vi "Dispense X Gallon at Y Flowrate.vi"(0 "Gallon Target":dbl=10.72, 1 "Equipment":T3={"MW100"="MW100", "AG34970"="A-34972A", "WT210"="A-34972A"}, 5 "GPM Target":dbl=3.0, 11 "Error In":errorcluster, 12 "Test Condition":T5=enum."SRK500,Station1,5GPM FR", 13 "Ctl Refnum":refnum<vi>) -> (6 "M*(Gallons)":dbl, 8 "ToutMax":dbl, 10 "ToutMin":dbl, 14 "POWER Ref":refnum<vi>, 15 "Error Out":errorcluster)   [LabVIEW 2013]
uses:
  Utility/Custom Pallet Controls/Chart.ctl
  Type Definitions/PowerElements.ctl
  Type Definitions/EquipReferences.ctl
  Type Definitions/HEWH Tank Indicator.ctl
  Type Definitions/TestedFlowratesScenarios.ctl
  Utility/Custom Pallet Controls/Timer.ctl
  Type Definitions/PowerData.ctl
  Type Definitions/User Controls.ctl
  Type Definitions/HEWH Output Information.ctl
  <vilib>/Platform/fileVersionInfo.llb/FileVersionInformation.ctl
  Type Definitions/Agilent Cluster.ctl
  Type Definitions/Draw Pattern Setup.ctl
  Type Definitions/PreDraw.ctl
  Type Definitions/Custom Test.ctl
  Type Definitions/Custom Test - Conditions.ctl
  Type Definitions/Termination Condition Cluster.ctl
  Utility/Custom Pallet Controls/DBL.ctl
  Type Definitions/ChannelSettings.ctl
  Type Definitions/Intellfaucet Mode.ctl
panel:
  out "Gather Data Timer":dbl format="%.2f"
  out "Loop Time":dbl
  out "PowerData":T1={"Voltage (Volts)"=236.2, "Current (Amps)"=17.749, "Power (Watts)"=4192.0, "WattHours (Wh)"=0.0, "TC Tree (AVG)"=0.0, "Flow Rate (GPM)"=0.0, "Gallons (Gal)"=0.0, "RTD Out (Deg F)"=0.0, "TC Down"=0.0}
  out "Elapsed Time":T2 format="%<%H:%M:%S>t"
  in  "Tab Control":enum32{"Page 1", "Page 2"}(tab)
  in  "Equipment 2":T3={"MW100"="COM1", "AG34970"="MW100", "WT210"="A-34972A"}
  out "Flow":dbl=3.8899999999999997
  out "String":string
  out "POWER":T4
  out "Dispensed Gallons":dbl
  in  "Gallon Target Value":dbl format="%#_13g"
  in  "GPM Target Value":dbl format="%#_13g"
  in  "Configuration":T5=enum."SRK500,Station1,5GPM FR"
  in  "OK":bool
  out "Tank Display":T6 {"TC6" format="%.2g"; "TIN" format="%.2g"; "TOUT" format="%.2g"; "Mean" format="%.2f"; "Std Dev" format="%.2f"; "TC5" format="%.2g"; "TC4" format="%.2g"; "TC3" format="%.2g"; "TC2" format="%.2g"; "TC1" format="%.2g"}
  out "Flow Chart":T7
  out "MW100":refnum<visa-resource-name>="MW100"
  out "Current Draw Start Time":dbl format="%.2f"
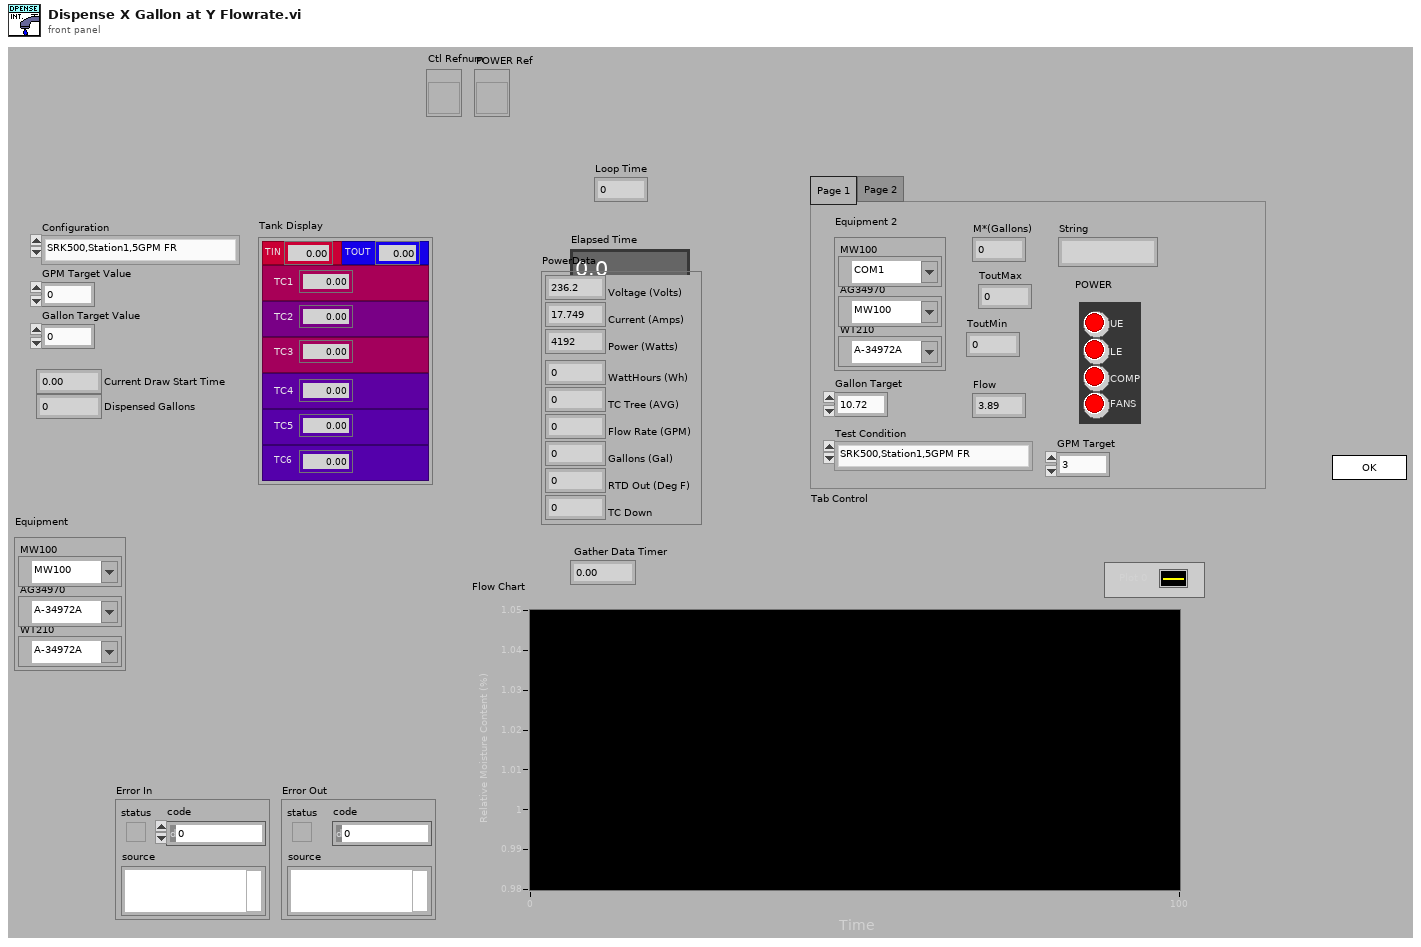
[diagram p1: front panel]
types:
  T1 = typedef "PowerData.ctl" = cluster{"Voltage (Volts)":dbl, "Current (Amps)":dbl, "Power (Watts)":dbl, "WattHours (Wh)":dbl, "TC Tree (AVG)":dbl, "Flow Rate (GPM)":dbl, "Gallons (Gal)":dbl, "RTD Out (Deg F)":dbl, "TC Down":dbl}
  T2 = typedef "Timer.ctl" = dbl
  T3 = typedef "EquipReferences.ctl" = cluster{"MW100":refnum<visa-resource-name>, "AG34970":refnum<visa-resource-name>, "WT210":refnum<visa-resource-name>}
  T4 = typedef "PowerElements.ctl" = cluster{"UE":bool, "LE":bool, "COMP":bool, "FANS":bool}
  T5 = typedef "TestedFlowratesScenarios.ctl" = enum16{"DRK500,Station1", "DRK375,Lab", "SRK500,Station1,5GPM FR", "DRK375,STATION3,1/2\"HOSE", "DRK500,Station1,downspout", "DRK375,Station3,thruEcocute", "DRK375,Station3,purge", "Build2,2B,Purge", "Global, Purge", "Global, Tank", "DRK250"}
  T6 = typedef "HEWH Tank Indicator.ctl" = cluster{"TC1-D":bool, "TC2-D":bool, "TC3-D":bool, "TC4-D":bool, "TC5-D":bool, "RTD_IN":bool, "RTDOUT":bool, "TC1":dbl, "TC2":dbl, "TC3":dbl, "TC4":dbl, "TC5":dbl, "TIN":dbl, "TOUT":dbl, "Std Dev":dbl, "Mean":dbl, "TC6-D":bool, "TC6":dbl}
  T7 = typedef "Chart.ctl" = dbl
  T8 = typedef "Intellfaucet Mode.ctl" = enum16{"Adjust Temp", "Adjust Flow", "Start Flow", "Stop Flow"}
  T9 = enum32{"invalid app kind", "Development System", "Run Time System", "Student Edition", "Embedded LabVIEW", "Evaluation", "Custom"}
  T10 = enum32{"Invalid", "Standard", "Closed", "Hidden", "Minimized", "Maximized"}
  T11 = typedef "User Controls.ctl" = cluster{"Main Power Control":bool, "Out VLV":enum8{"CLOSE", "OPEN"}, "Expansion Tank?":bool, "In VLV":enum8{"OPEN", "CLOSE"}, "Drain VLV":enum8{"OPEN", "CLOSE"}, "Flow Totalizer Control":bool, "Intellifaucet Temperature":dbl, "Percent Flow":dbl, "Safe Mode":bool, "In VLV B":enum8{"OPEN", "CLOSE"}, "Drain VLV B":enum8{"OPEN", "CLOSE"}, "Out VLV B":enum8{"CLOSE", "OPEN"}, "In VLV C":enum8{"OPEN", "CLOSE"}, "Drain VLV C":enum8{"OPEN", "CLOSE"}, "Out VLV C":enum8{"CLOSE", "OPEN"}, "In VLV D":enum8{"OPEN", "CLOSE"}, "Drain VLV D":enum8{"OPEN", "CLOSE"}, "Out VLV D":enum8{"CLOSE", "OPEN"}, "GEA2?":bool, "Use Agilent?":bool, "Valve Set A":enum16{"Heating", "Purge", "Resting", "Draw"}, "Valve Set B":enum16{"Heating", "Purge", "Resting", "Draw"}, "Valve Set C":enum16{"Heating", "Purge", "Resting", "Draw"}, "Valve Set D":enum16{"Heating", "Purge", "Resting", "Draw"}}
  T12 = typedef "HEWH Output Information.ctl" = cluster{"TR Number:":string, "Lab ID:":string, "Calibration Array":string[][], "Test Number:":string, "Model:":string, "Serial Number:":string, "Build:":string, "Ambient Temp SetPoint:":string, "Test Station:":string, "Frequency:":string, "Ambient RH:":string, "Comments:":string, "Technician:":string, "Engineer:":string, "Date:":string, "Version:":string, "Computer:":string, "Filename":string, "Heating Mode":string, "FileVersionInfo":T13, "File Initialization Array":string[][], "File Path":path, "Computer IP Address:":string, "Agilent Channel List":string, "Agilent Cluster Array":T14[], "Calibration Coefficients":dbl[][], "Agilent Raw Cluster Array":T14[], "Data Table":string[][], "RLT Station?":bool, "Scan Rate Adjust":dbl, "Start Gallons":dbl, "Last GPM Reading":dbl, "PowerData":T1, "Draw Count":i32, "Draw Patten Setup":T15, "Draw Until Condition":T4, "TC Tree":dbl[], "Starting Temp Decline Temp":dbl, "Full Data Table":string[][], "Max RTD Temp\nDuring Draw":dbl, "Min RTD Temp\nDuring Draw":dbl, "RTD Max Min Array":dbl[][], "Draw Start Time":dbl, "Draw Statistics":dbl[][], "Last Temp Reading":dbl, "Custom Test Array":T17[], "Delay Start Time":dbl, "Condition Cluster Output":T19}
  T13 = typedef "FileVersionInformation.ctl" = cluster{"FileVersion":string, "ProductName":string, "InternalName":string, "CompanyName":string, "LegalCopyright":string, "FileDescription":string}
  T14 = typedef "Agilent Cluster.ctl" = cluster{"Label":string, "Agilent Channel":string, "Panel ID":string, "Source":string, "Temperature":dbl}
  T15 = typedef "Draw Pattern Setup.ctl" = cluster{"Dispense Times":dbl[], "Total Gallons Schedule":dbl[], "Flow Rate Schedule ":dbl[], "Incoming Water Temperature":dbl[], "PreDraw Pattern":dbl[][], "Repeat":bool, "24 Hour PreDraw":T16}
  T16 = typedef "PreDraw.ctl" = enum16{"Zero Pre-Draws", "One Pre- Draws", "Two Pre-Draws", "Three Pre-Draws", "High Usage Pre-Draw", "Medium Usage Pre-Draw", "Low Usage Pre-Draw"}
  T17 = typedef "Custom Test.ctl" = cluster{"Custom Test Value":dbl, "Flow Rate (GPM)":dbl, "Incoming Water  Temperature ":dbl, "Action Type":T18}
  T18 = typedef "Custom Test - Conditions.ctl" = enum16{"", "Draw - Elapsed Time (sec)", "Draw - Gallon Target", "Draw - Until Comp", "Draw - Until Comp & Fan", "Draw - Until LE", "Draw - Until UE", "Draw - Any Heat Source", "Draw - Until RTD Out Temp", "Draw - Until RTD Out Temp Reduction", "Draw - Until Mean Tank Temp", "Wait - Cutout", "Wait - Comp ON", "Wait - Comp & Fan ON", "Wait - Comp OFF", "Wait - Comp & Fan OFF", "Wait - LE ON", "Wait - LE OFF", "Wait - UE ON", "Wait - UE OFF", "Wait - Elapsed Time (sec)", "Wait - RTD Out Temp", "Wait - RTD Out Temp Reduction", "Wait - Mean Tank Temp", "Terminate - Comp ON", "Terminate - Comp & Fan ON", "Terminate - Comp OFF", "Terminate - Comp & Fan OFF", "Terminate - LE ON", "Terminate - LE OFF", "Terminate - UE ON", "Terminate - UE OFF", "Terminate - RTD Out Temp", "Terminate - Mean Tank Temp", "Terminate - UE or LE ON", "Terminate - UE or LE OFF", "Terminate - Cutout", "Repeat"}
  T19 = typedef "Termination Condition Cluster.ctl" = cluster{"Decrease RTD Output\nTemperature Bool":bool, "RTD Out Temperature Bool":bool, "Use Time Bool":bool, "RTD Out Temperature":T20, "Decrease Outlet Temperature By (RTD Out)":T20, "Time (Seconds)":T20, "Draw Until Condition":T4, "Start Draw Until Specific Bool":bool, "Return Output Bool":bool, "Draw Until Any Heat Bool":bool, "Mean Tank Temperature Bool":bool, "Mean Tank Temperature":T20, "Comp OFF":bool, "Comp & Fan OFF":bool, "UE OFF":bool, "LE OFF":bool}
  T20 = typedef "DBL.ctl" = dbl
  T21 = cluster{"Core":cluster{"Current VI Reference":refnum<vi>, "Close Panel on Exit?":bool}, "Equipment":T3, "User Controls":T11, "FileInit Cluster":T12, "PowerData":T1, "Last GPM Reading":dbl, "GPM Target Value":dbl, "Gallon Target Value":dbl, "Start Gallons":dbl}
  T22 = cluster{"Current VI Reference":refnum<vi>, "Close Panel on Exit?":bool}
  T23 = typedef "ChannelSettings.ctl" = u32
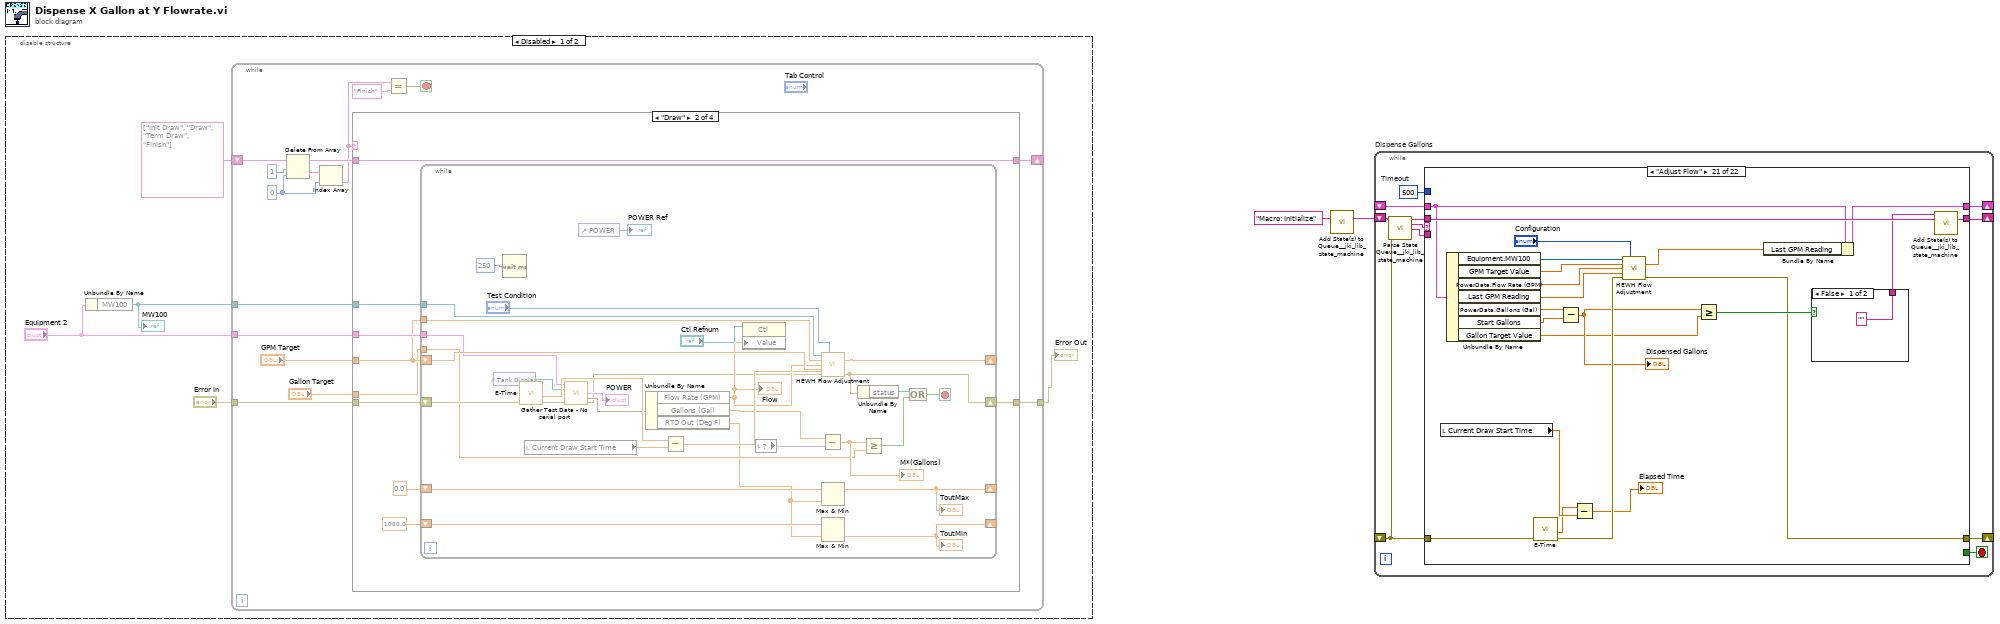
[diagram p0: block diagram]
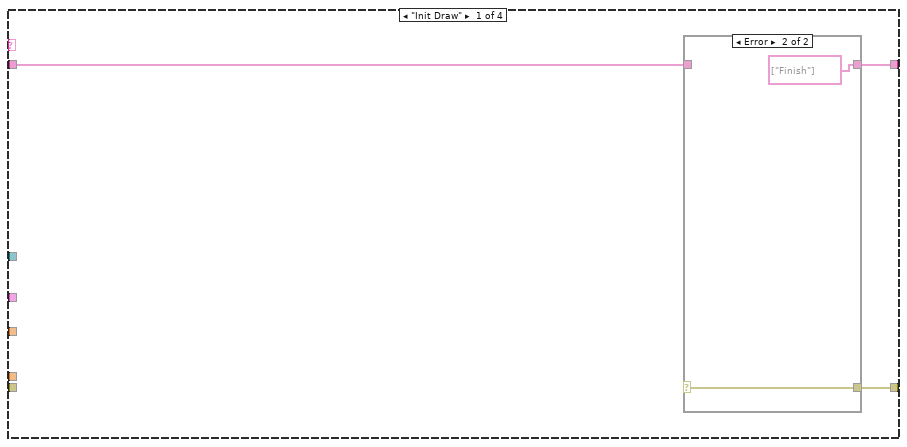
[diagram p2: hidden frame]
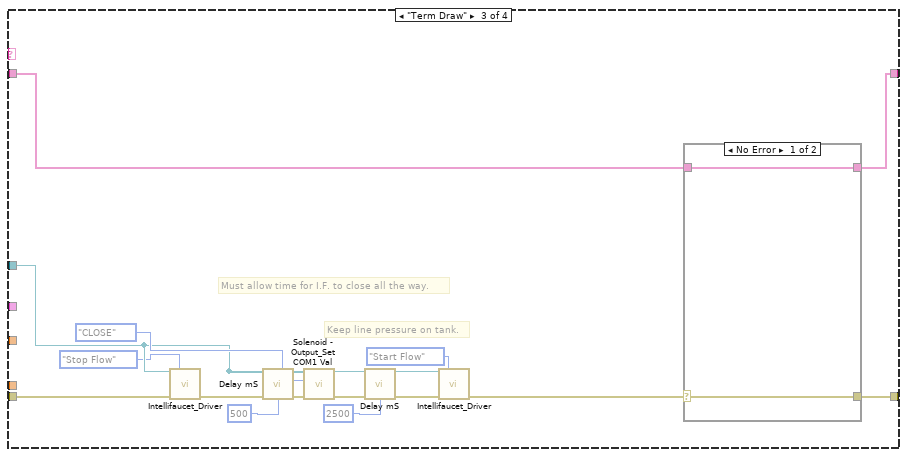
[diagram p4: hidden frame]
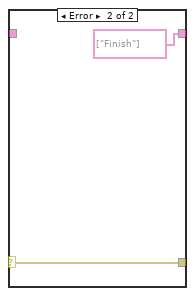
[diagram p5: hidden frame]
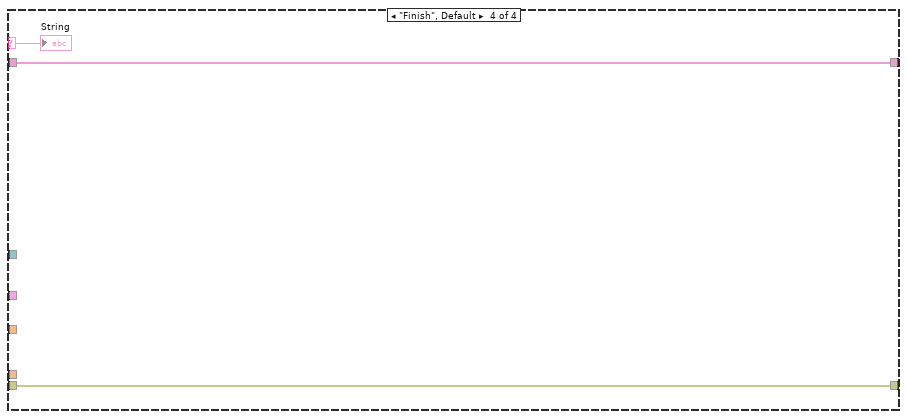
[diagram p6: hidden frame]
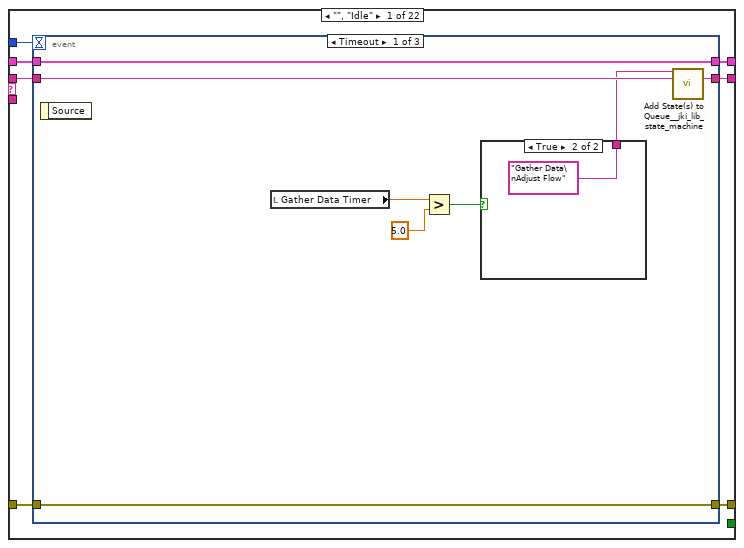
[diagram p8: hidden frame]
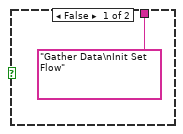
[diagram p9: hidden frame]
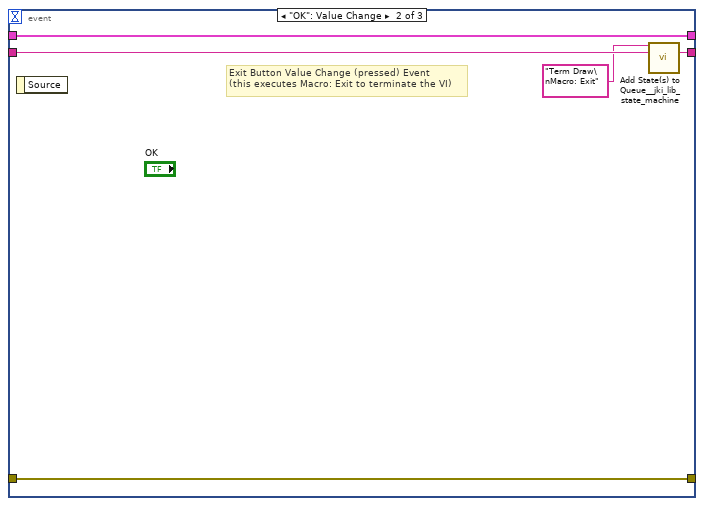
[diagram p10: hidden frame]
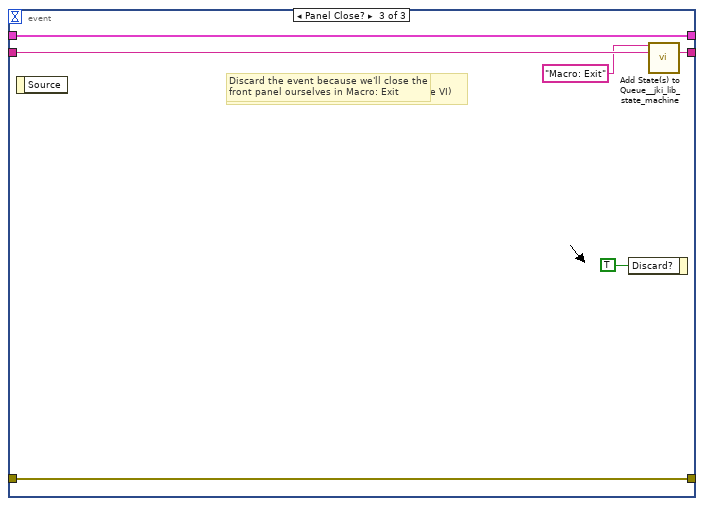
[diagram p11: hidden frame]
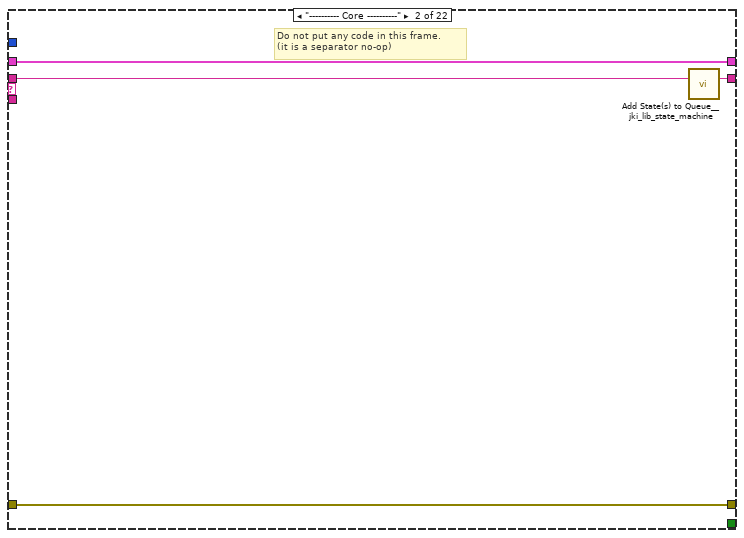
[diagram p12: hidden frame]
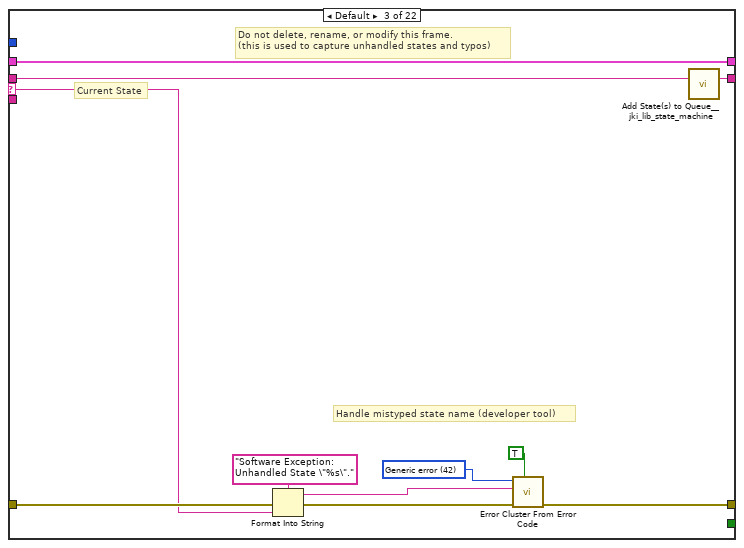
[diagram p13: hidden frame]
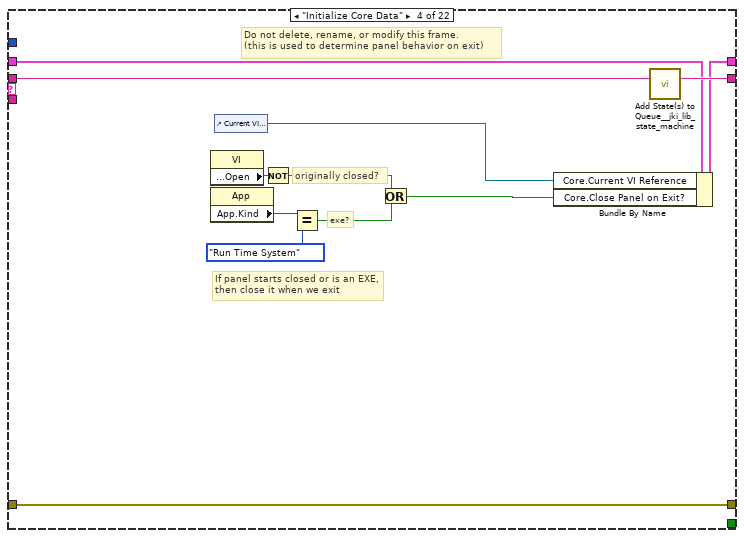
[diagram p14: hidden frame]
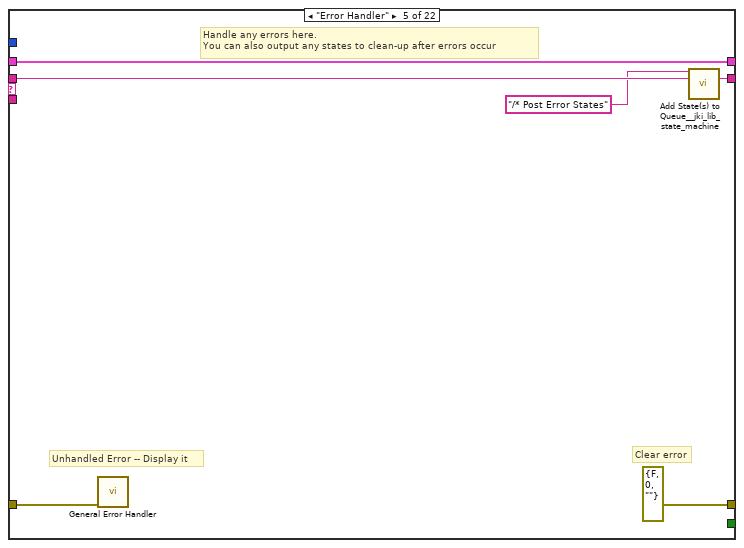
[diagram p15: hidden frame]
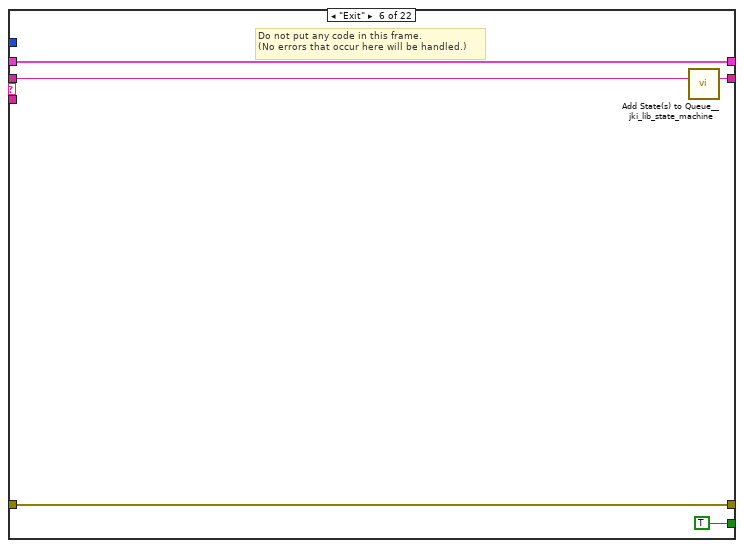
[diagram p16: hidden frame]
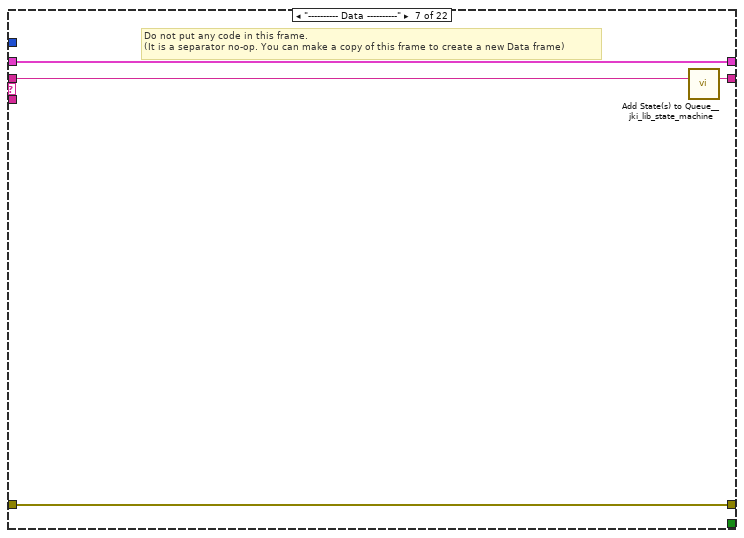
[diagram p17: hidden frame]
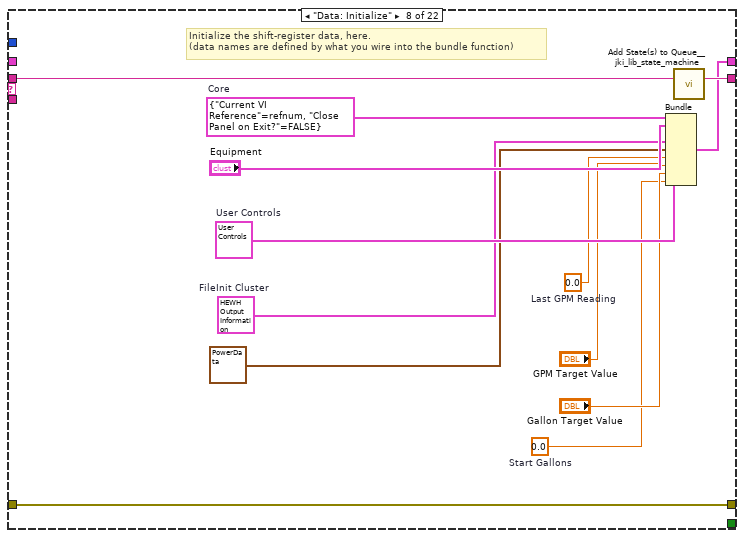
[diagram p18: hidden frame]
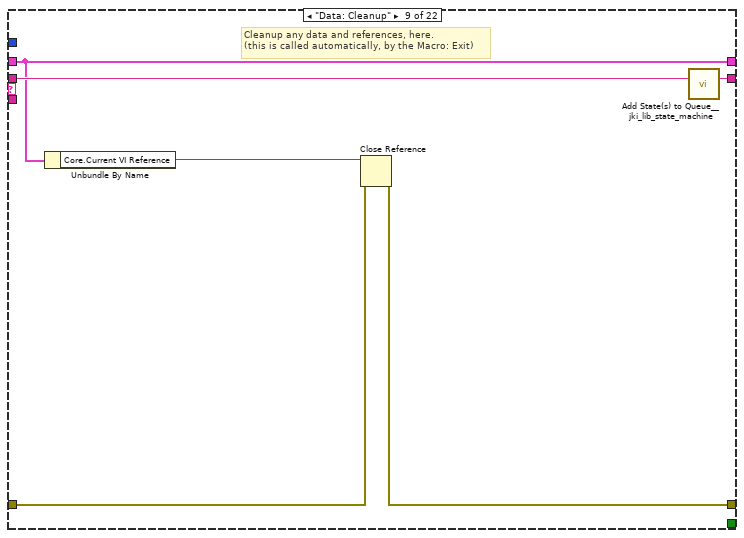
[diagram p19: hidden frame]
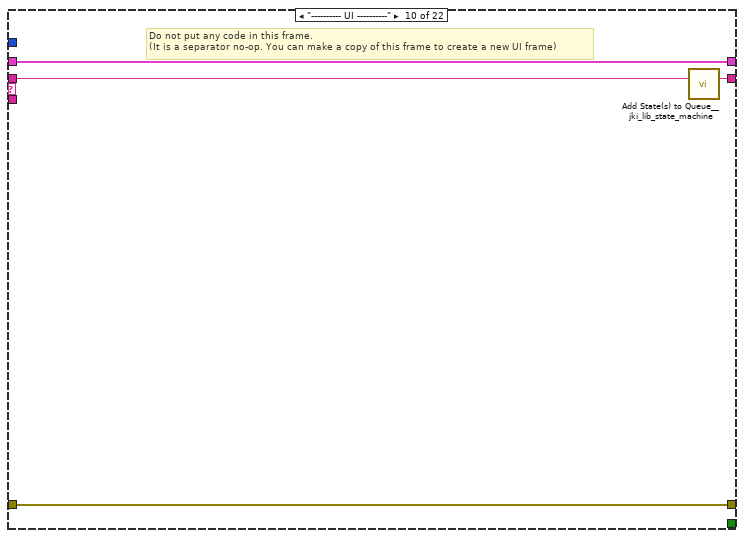
[diagram p20: hidden frame]
diagram:
  n1 = disable-structure shown="Disabled" {
    frame Disabled {
      n2 = Unbundle By Name("Equipment 2") -> ("MW100"=w5:refnum<visa-resource-name>)
      "MW100" <- w5
      n3 = while {
        tunnel: "Error In" -> [w22]
        tunnel: "Equipment 2" -> [w16]
        tunnel: w5 -> [w15]
        tunnel: [w14] -> w3
        shift-right: [w12] -> _
        shift-left: string[] ["Init Draw", "Draw", "Term Draw", "Finish"] ("array") -> [w17]
        stop <- w9 stop-if-true
        w19 = 0 ("index")
        n4 = Delete From Array(array=w17, length=1, index=w19) -> (deleted portion=w20:string[], array with subset deleted=w18:string[])
        n5 = Index Array(array=w20, index=w19) -> (element=w11:string)
        n6 = case shown="\"Draw\"" w11 {
          selector: w11 -> [_ _ _ w92]
          tunnel: [w24 w36 w83 w90] -> w12
          tunnel: w18 -> [w25 w36 w84 w90]
          tunnel: [w23 w38 w82 w91] -> w14
          tunnel: w22 -> [_ w35 w81 w91]
          tunnel: w16 -> [_ w34 _ _]
          tunnel: w15 -> [_ w33 w79 _]
          tunnel: "GPM Target" -> [_ w31 _ _]
          tunnel: "Gallon Target" -> [_ w30 _ _]
          frame "Init Draw" {
            n7 = case shown="Error" {
              selector: _ -> [w26 w29]
              tunnel: [w27 string[] ["Finish"] ("States")] -> w24
              tunnel: w25 -> [w27 _]
              tunnel: [w26 w29] -> w23
              frame No Error {
              }
              frame Error {
              }
            }
          }
          frame "Draw" {
            n8 = while {
              shift-right: [w62] -> w38
              shift-left: w35 -> [w51]
              shift-right: [w68] -> _
              shift-left: w31 -> [w69]
              shift-right: [w58] -> _
              shift-left: 0.0 ("GPM") -> [w59]
              tunnel: w34 -> [w40]
              tunnel: w33 -> [w55]
              shift-right: [w57] -> _
              shift-left: 1000.0 -> [w56]
              tunnel: w31 -> [w52]
              tunnel: w30 -> [w50]
              stop <- w70 stop-if-true
              n9 = control-ref of="Tank Display"() -> (w48:refnum<vi>)
              n10 = Wait (ms)(milliseconds to wait=u32 250) -> ()  [unwired: 1 out]
              n11 = call "E-Time.vi"("error in (no error)"=w51) -> ("error out"=w66:errorcluster, "Elapsed Time (sec)"=w64:dbl)  [unwired: 8 in, 1 out]
              n12 = local read "Current Draw Start Time"() -> (w54:dbl)
              n13 = call "Gather Test Data - No serial port.vi"("Equipment"=w40, "Tank Display Ref"=w48, "error in (no error)"=w66) -> ("POWER"=→"POWER":T4, "PowerData"=w45:T1, "error out"=w41:errorcluster)  [unwired: 8 in, 2 out]
              n14 = control-ref of="POWER"() -> (→"POWER Ref":refnum<vi>)
              n15 = Unbundle By Name(w45) -> ("Flow Rate (GPM)"=w44:dbl, "Gallons (Gal)"=w42:dbl, "RTD Out (Deg F)"=w43:dbl)
              "Flow" <- w44
              n16 = Subtract(x=w64, y=w54) -> (x-y=w63:dbl)
              n17 = property class="Ctl"(reference="Ctl Refnum", "Value"=w44) -> ()  [unwired: 1 in, 2 out]
              n18 = local read item#-1() -> (w60)
              n19 = Subtract(x=w42, y=w60) -> (x-y=w53:dbl)
              "M*(Gallons)" <- w53
              n20 = call "HEWH Flow Adjustment.vi"("VISA session"=w55, "Configuration"="Test Condition", "GPM Target(3)"=w52, "GPM reading"=w44, "New GPM Reading \nfrom last adjustment"=w69, "Error In"=w41, 12:w63) -> ("Flow rate setting Out"=w68:dbl, "Error Out"=w62:errorcluster)  [unwired: 6 in, 1 out]
              n21 = Max & Min(x=w59, y=w43) -> (max(x,y)=w58:dbl)  [unwired: 1 out]
              "ToutMax" <- w58
              n22 = Max & Min(x=w56, y=w43) -> (min(x,y)=w57:dbl)  [unwired: 1 out]
              "ToutMin" <- w57
              n23 = Unbundle By Name(w62) -> ("status"=w67:bool)
              n24 = Greater Or Equal?(x=w53, y=w50) -> (x >= y?=w65:bool)
              n25 = Compound Arithmetic op=OR(w67, w65) -> (w70:bool)
            }
          }
          frame "Term Draw" {
            # "Must allow time for I.F. to close all the way."
            # "Keep line pressure on tank."
            n26 = call "Intellifaucet_Driver.vi"("VISA session"=w79, "Mode"=Intellfaucet_Mode."Stop Flow", "Error In"=w81) -> ("Error Out"=w77:errorcluster)  [unwired: 11 in, 1 out]
            n27 = call "Delay mS.vi"("Error In"=w77, "milliseconds to wait"=u32 500) -> ("Error Out"=w76:errorcluster)  [unwired: 13 in]
            n28 = call "Solenoid - Output_Set COM1 Val.vi"("Error In"=w76, "OPEN CLOSE"=enum8{"CLOSE", "OPEN"}."CLOSE", "VISA session"=w79) -> ("Error Out"=w72:errorcluster)  [unwired: 7 in, 1 out]
            n29 = call "Delay mS.vi"("Error In"=w72, "milliseconds to wait"=u32 2500) -> ("Error Out"=w71:errorcluster)  [unwired: 13 in]
            n30 = call "Intellifaucet_Driver.vi"("VISA session"=w79, "Mode"=Intellfaucet_Mode."Start Flow", "Error In"=w71) -> ("Error Out"=w80:errorcluster)  [unwired: 11 in, 1 out]
            n31 = case shown="No Error" w80 {
              selector: w80 -> [w86 w89]
              tunnel: [w87 string[] ["Finish"] ("States")] -> w83
              tunnel: w84 -> [w87 _]
              tunnel: [w86 w89] -> w82
              frame No Error {
              }
              frame Error {
              }
            }
          }
          frame "Finish", Default {
            "String" <- w92
          }
        }
        n32 = Equal?(x=w11, y="Finish") -> (x = y?=w9:bool)
      }
      "Error Out" <- w3
    }
    frame Enabled {
    }
  }
  n33 = call <vilib>:"Add State(s) to Queue__jki_lib_state_machine.vi"("State(s) in (\"\")"="Macro: Initialize") -> ("States Out"=w2:string)  [unwired: 14 in]
  n34 = while "Dispense Gallons" {
    shift-right: [w96] -> _
    shift-left: _ -> [w95]
    shift-right: [w99] -> _
    shift-left: _ -> [w93]
    shift-right: [w98] -> _
    shift-left: w2 -> [w100]
    stop <- w97 stop-if-true
    w94 = 500  # Timeout
    n35 = call <vilib>:"Parse State Queue__jki_lib_state_machine.vi"("State Queue"=w100, "Error In (no error)"=w93) -> ("Remaining States"=w102:string, "Current State"=w103:string, "Arguments"=w101:string)  [unwired: 11 in]
    n36 = case shown="\"Adjust Flow\"" w103 {
      selector: w103 -> [_ _ w136 _ _ _ _ _ _ _ _ _ _ _ _ _ _ _ _ _ _ _]
      tunnel: w102 -> [w110 w135 w140 w158 w164 w169 w173 w186 w192 w196 w200 w206 w217 w243 w248 w258 w262 w290 w306 w319 w341 w358]
      tunnel: w101 -> [_ _ _ _ _ _ _ _ _ _ _ w201 w211 _ _ _ _ _ _ _ _ _]
      tunnel: w95 -> [w108 w132 w138 w149 w161 w167 w170 _ w187 w193 w198 w204 w213 w240 w245 w255 w259 w265 w299 w315 w323 w345]
      tunnel: [w107 w133 w142 w155 errorcluster {"status"=FALSE, "code"=0, "source"=""} ("error out") w166 w171 w183 w188 w194 w197 w202 w214 w241 w246 w256 w260 w266 w301 w317 w320 w346] -> w99
      tunnel: w93 -> [w106 w133 w141 w155 w160 w166 w171 w183 w189 w194 w197 w203 w215 w241 w246 w256 w260 w267 w296 w313 w334 w347]
      tunnel: [w109 w134 w139 w157 w163 w168 w172 w185 w191 w195 w199 w205 w216 w242 w247 w257 w261 w289 w305 w318 w340 w357] -> w98
      tunnel: [_ _ _ _ _ TRUE _ _ _ _ _ _ _ _ _ _ _ _ _ _ _ _] -> w97
      tunnel: [w105 w132 w138 w156 w161 w167 w170 w184 w187 w193 w198 w204 w213 w240 w245 w255 w259 w264 w298 w316 w322 w345] -> w96
      tunnel: w94 -> [w104 _ _ _ _ _ _ _ _ _ _ _ _ _ _ _ _ _ _ _ _ _]
      frame "", "Idle" {
        n37 = event shown="[0] Timeout" {
          selector: _ -> [_ _ _]
          dyn-events: _ -> [_ _ _]
          timeout: w104 -> [_ _ _]
          tunnel: w110 -> [w118 w125 w131]
          tunnel: [w117 w124 w130] -> w109
          tunnel: w108 -> [w115 w122 w128]
          tunnel: [w116 w123 w129] -> w107
          tunnel: w106 -> [w116 w123 w129]
          tunnel: [w115 w122 w128] -> w105
          event Timeout {
            n38 = event-data() -> ()  [unwired: 1 in, 1 out]
            n39 = local read "Gather Data Timer"() -> (w113:dbl)
            n40 = Greater?(x=w113, y=5.0) -> (0:w111:bool)
            n41 = case shown="True" w111 {
              tunnel: ["Gather Data\nInit Set Flow" "Gather Data\nAdjust Flow"] -> w114
              frame False {
              }
              frame True {
              }
            }
            n42 = call <vilib>:"Add State(s) to Queue__jki_lib_state_machine.vi"("State(s) in Front (\"\")"=w114, "State(s) in (\"\")"=w118) -> ("States Out"=w117:string)  [unwired: 13 in]
          }
          event "OK": Value Change {
            # "Exit Button Value Change (pressed) Event\n(this executes Macro: Exit to terminate the VI)"
            n43 = event-data() -> ()  [unwired: 1 in, 1 out]
            n44 = call <vilib>:"Add State(s) to Queue__jki_lib_state_machine.vi"("State(s) in Front (\"\")"="Term Draw\nMacro: Exit", "State(s) in (\"\")"=w125) -> ("States Out"=w124:string)  [unwired: 13 in]
          }
          event Panel Close? {
            # "Discard the event because we'll close the front panel ourselves in Macro: Exit"
            # "Close Panel button (pressed) Event\n(this executes Macro: Exit to terminate the VI)"
            n45 = event-data() -> ()  [unwired: 1 in, 1 out]
            n46 = event-data("Discard?"=TRUE) -> ()  [unwired: 1 in, 1 out]
            n47 = call <vilib>:"Add State(s) to Queue__jki_lib_state_machine.vi"("State(s) in Front (\"\")"="Macro: Exit", "State(s) in (\"\")"=w131) -> ("States Out"=w130:string)  [unwired: 13 in]
          }
        }
      }
      frame "---------- Core ----------" {
        # "Do not put any code in this frame.\n(it is a separator no-op)"
        n48 = call <vilib>:"Add State(s) to Queue__jki_lib_state_machine.vi"("State(s) in (\"\")"=w135) -> ("States Out"=w134:string)  [unwired: 14 in]
      }
      frame Default {
        w145 = 42 items=["No error", "Argument error", "Memory is full", "Out of zone", "End of file", "File already open", "Generic file I/O error", "File not found", "File permission error", "Disk is full", "Duplicate path", "Too many files open", "System feature not enabled", "Resource file not found", "Cannot add resource", "Resource not found", "Image not found", "Image memory error", "Pen does not exist", "Config type invalid", "Config token not found", "Config parse error", "Config memory error", "Bad external code format", "Bad external code offset", "External code not present", "Null window", "Destroy window error", "Null menu", "Print aborted", "Bad print record", "Print driver error", "Windows error during printing", "Memory error during printing", "Print dialog error", "Generic print error", "Invalid device refnum", "Device not found", "Device parameter error", "Device unit error", "Cannot open device", "Device call aborted", "Generic error", "Cancelled by user", "Object ID too low", "Object ID too high", "Object not in heap", "Unknown heap", "Unknown object (invalid DefProc)", "Unknown object (DefProc not in table)", "Message out of range", "Invalid (null) method", "Unknown message", "Manager call not supported", "Bad address", "Network operation in progress", "Network operation timed out", "Connection is busy", "Network attribute not supported", "Network error", "Address in use", "System out of memory", "Connection aborted", "Connection refused", "Not connected", "Already connected", "Connection closed", "Initialization error (interapplication manager)", "Bad occurrence", "Wait on unbound occurrence handler", "Occurrence queue overflow", "Datalog type conflict", "Unused", "Unrecognized type (interapplication manager)", "Memory corrupt", "Failed to make temporary DLL", "Old CIN version", "Drag socket not found", "Failed to load drop-object", "Failed to register OLE object", "Failed to release OLE object", "Format specifier type mismatch", "Unknown format specifier", "Too few format specifiers", "Too many format specifiers", "Scan failed", "Newer CIN version", "Error converting to variant", "Runtime menu error", "Password tampered", "Variant attribute not found", "Incompatible variant data type", "Event data is not available", "Event Store is not present", "Occurrence is not found", "Event Queue is not created", "Event info is not available", "Refnum passed is NULL", "Error retrieving Class GUID", "Error retrieving CoClass GUID", "Error retrieving TypeLib GUID.", "Bad built application magic bytes.", "Specific driver is different from the specific driver associated with the Logical Name.", "There is no session opened to the class driver.", "Max Error", "MAX - Error with config objects", "MAX - Error loading configuration", "MAX - Group not supported"]
        # "Current State"
        # "Do not delete, rename, or modify this frame.\n(this is used to capture unhandled states and typos)"
        # "Handle mistyped state name (developer tool)"
        n49 = Format Into String(format string="Software Exception: Unhandled State \"%s\"." ("message"), error in=w141, w136) -> (resulting string=w144:string, error out=w143:errorcluster)  [unwired: 1 in]
        n50 = call <vilib>:"Error Cluster From Error Code.vi"("show call chain? (False)"=TRUE, "error in (no error)"=w143, "error message (\"\")"=w144, "error code (0)"=w145) -> ("error out"=w142:errorcluster)  [unwired: 5 in]
        n51 = call <vilib>:"Add State(s) to Queue__jki_lib_state_machine.vi"("State(s) in (\"\")"=w140) -> ("States Out"=w139:string)  [unwired: 14 in]
      }
      frame "Initialize Core Data" {
        # "Do not delete, rename, or modify this frame.\n(this is used to determine panel behavior on exit)"
        # "originally closed?"
        # "exe?"
        # "If panel starts closed or is an EXE, then close it when we exit"
        n52 = property class="VI"() -> ("Front Panel.Open"=w154:bool)  [unwired: 2 in, 2 out]
        n53 = property class="App"() -> ("App.Kind"=w153:T9)  [unwired: 2 in, 2 out]
        n54 = control-ref of="Current VI Reference"() -> (w147:refnum<vi>)
        n55 = Not(x=w154) -> (.not. x?=w151:bool)
        n56 = Equal?(x=w153, y=T9."Run Time System" ("Application:Kind")) -> (x = y?=w150:bool)
        n57 = Or(x=w151, y=w150) -> (x .or. y?=w148:bool)
        n58 = Bundle By Name(cluster=w149, "Core.Current VI Reference"=w147, "Core.Close Panel on Exit?"=w148) -> (w156:T21)
        n59 = call <vilib>:"Add State(s) to Queue__jki_lib_state_machine.vi"("State(s) in (\"\")"=w158) -> ("States Out"=w157:string)  [unwired: 14 in]
      }
      frame "Error Handler" {
        # "Unhandled Error -- Display it"
        # "Handle any errors here.\nYou can also output any states to clean-up after errors occur"
        # "Clear error"
        n60 = call <vilib>:"General Error Handler.vi"("error in (no error)"=w160) -> ()  [unwired: 10 in, 5 out]
        n61 = call <vilib>:"Add State(s) to Queue__jki_lib_state_machine.vi"("State(s) in Front (\"\")"="/* Post Error States", "State(s) in (\"\")"=w164) -> ("States Out"=w163:string)  [unwired: 13 in]
      }
      frame "Exit" {
        # "Do not put any code in this frame.\n(No errors that occur here will be handled.)"
        n62 = call <vilib>:"Add State(s) to Queue__jki_lib_state_machine.vi"("State(s) in (\"\")"=w169) -> ("States Out"=w168:string)  [unwired: 14 in]
      }
      frame "---------- Data ----------" {
        # "Do not put any code in this frame.\n(It is a separator no-op. You can make a copy of this frame to create a new Data frame)"
        n63 = call <vilib>:"Add State(s) to Queue__jki_lib_state_machine.vi"("State(s) in (\"\")"=w173) -> ("States Out"=w172:string)  [unwired: 14 in]
      }
      frame "Data: Initialize" {
        w174 = 0.0  # Start Gallons
        w177 = 0.0  # Last GPM Reading
        w179 = T12 {"TR Number:"="", "Lab ID:"="", "Calibration Array"=[], "Test Number:"="", "Model:"="", "Serial Number:"="", "Build:"="", "Ambient Temp SetPoint:"="", "Test Station:"="", "Frequency:"="", "Ambient RH:"="", "Comments:"="", "Technician:"="", "Engineer:"="", "Date:"="", "Version:"="", "Computer:"="", "Filename"="", "Heating Mode"="", "FileVersionInfo"={"FileVersion"="", "ProductName"="", "InternalName"="", "CompanyName"="", "LegalCopyright"="", "FileDescription"=""}, "File Initialization Array"=[], "File Path"=path "", "Computer IP Address:"="", "Agilent Channel List"="", "Agilent Cluster Array"=[], "Calibration Coefficients"=[], "Agilent Raw Cluster Array"=[], "Data Table"=[], "RLT Station?"=FALSE, "Scan Rate Adjust"=0.0, "Start Gallons"=0.0, "Last GPM Reading"=0.0, "PowerData"={"Voltage (Volts)"=0.0, "Current (Amps)"=0.0, "Power (Watts)"=0.0, "WattHours (Wh)"=0.0, "TC Tree (AVG)"=0.0, "Flow Rate (GPM)"=0.0, "Gallons (Gal)"=0.0, "RTD Out (Deg F)"=0.0, "TC Down"=0.0}, "Draw Count"=0, "Draw Patten Setup"={"Dispense Times"=[], "Total Gallons Schedule"=[], "Flow Rate Schedule "=[], "Incoming Water Temperature"=[], "PreDraw Pattern"=[], "Repeat"=FALSE, "24 Hour PreDraw"=enum."Zero Pre-Draws"}, "Draw Until Condition"={"UE"=FALSE, "LE"=FALSE, "COMP"=FALSE, "FANS"=FALSE}, "TC Tree"=[], "Starting Temp Decline Temp"=0.0, "Full Data Table"=[], "Max RTD Temp\nDuring Draw"=0.0, "Min RTD Temp\nDuring Draw"=0.0, "RTD Max Min Array"=[], "Draw Start Time"=0.0, "Draw Statistics"=[], "Last Temp Reading"=0.0, "Custom Test Array"=[], "Delay Start Time"=0.0, "Condition Cluster Output"={"Decrease RTD Output\nTemperature Bool"=FALSE, "RTD Out Temperature Bool"=FALSE, "Use Time Bool"=FALSE, "RTD Out Temperature"=0.0, "Decrease Outlet Temperature By (RTD Out)"=0.0, "Time (Seconds)"=0.0, "Draw Until Condition"={"UE"=FALSE, "LE"=FALSE, "COMP"=FALSE, "FANS"=FALSE}, "Start Draw Until Specific Bool"=FALSE, "Return Output Bool"=FALSE, "Draw Until Any Heat Bool"=FALSE, "Mean Tank Temperature Bool"=FALSE, "Mean Tank Temperature"=0.0, "Comp OFF"=FALSE, "Comp & Fan OFF"=FALSE, "UE OFF"=FALSE, "LE OFF"=FALSE}}  # FileInit Cluster
        w180 = T11 {"Main Power Control"=FALSE, "Out VLV"=enum."CLOSE", "Expansion Tank?"=FALSE, "In VLV"=enum."OPEN", "Drain VLV"=enum."OPEN", "Flow Totalizer Control"=FALSE, "Intellifaucet Temperature"=0.0, "Percent Flow"=0.0, "Safe Mode"=FALSE, "In VLV B"=enum."OPEN", "Drain VLV B"=enum."OPEN", "Out VLV B"=enum."OPEN", "In VLV C"=enum."CLOSE", "Drain VLV C"=enum."OPEN", "Out VLV C"=enum."OPEN", "In VLV D"=enum."CLOSE", "Drain VLV D"=enum."OPEN", "Out VLV D"=enum."OPEN", "GEA2?"=FALSE, "Use Agilent?"=FALSE, "Valve Set A"=enum."Heating", "Valve Set B"=enum."Heating", "Valve Set C"=enum."Heating", "Valve Set D"=enum."Heating"}  # User Controls
        w182 = T22 {"Current VI Reference"=refnum, "Close Panel on Exit?"=FALSE}  # Core
        # "Initialize the shift-register data, here.\n(data names are defined by what you wire into the bundle function)"
        n64 = Bundle("Core"=w182, "Equipment"="Equipment", "User Controls"=w180, "FileInit Cluster"=w179, "PowerData"=T1 {"Voltage (Volts)"=-1.0, "Current (Amps)"=-1.0, "Power (Watts)"=-1.0, "WattHours (Wh)"=-1.0, "TC Tree (AVG)"=0.0, "Flow Rate (GPM)"=0.0, "Gallons (Gal)"=0.0, "RTD Out (Deg F)"=0.0, "TC Down"=0.0}, "Last GPM Reading"=w177, "GPM Target Value"="GPM Target Value", "Gallon Target Value"="Gallon Target Value", "Start Gallons"=w174) -> (w184:T21)  [unwired: 1 in]
        n65 = call <vilib>:"Add State(s) to Queue__jki_lib_state_machine.vi"("State(s) in (\"\")"=w186) -> ("States Out"=w185:string)  [unwired: 14 in]
      }
      frame "Data: Cleanup" {
        # "Cleanup any data and references, here.\n(this is called automatically, by the Macro: Exit)"
        n66 = Unbundle By Name(w187) -> ("Core.Current VI Reference"=w190:refnum<vi>)
        n67 = Close Reference(reference=w190, error in (no error)=w189) -> (error out=w188:errorcluster)
        n68 = call <vilib>:"Add State(s) to Queue__jki_lib_state_machine.vi"("State(s) in (\"\")"=w192) -> ("States Out"=w191:string)  [unwired: 14 in]
      }
      frame "---------- UI ----------" {
        # "Do not put any code in this frame.\n(It is a separator no-op. You can make a copy of this frame to create a new UI frame)"
        n69 = call <vilib>:"Add State(s) to Queue__jki_lib_state_machine.vi"("State(s) in (\"\")"=w196) -> ("States Out"=w195:string)  [unwired: 14 in]
      }
      frame "UI: Initialize" {
        # "Initialize the User Interface, here.\n(this is called automatically, by the Macro: Init)"
        n70 = call <vilib>:"Add State(s) to Queue__jki_lib_state_machine.vi"("State(s) in (\"\")"=w200) -> ("States Out"=w199:string)  [unwired: 14 in]
      }
      frame "UI: Cursor Set" {
        # "Argument"
        # "Set and Unset Cursor Busy.\n(Usage: \"UI: Cursor Set >> Busy|Idle\")"
        n71 = case shown="\"Idle\", Default" w201 {
          tunnel: w203 -> [w208 w210]
          tunnel: [w207 w209] -> w202
          frame "Idle", Default {
            n72 = call <vilib>:"Unset Busy.vi"("error in (no error)"=w208) -> ("error out"=w207:errorcluster)  [unwired: 10 in]
          }
          frame "Busy" {
            n73 = call <vilib>:"Set Busy.vi"("error in (no error)"=w210) -> ("error out"=w209:errorcluster)  [unwired: 9 in, 1 out]
          }
        }
        n74 = call <vilib>:"Add State(s) to Queue__jki_lib_state_machine.vi"("State(s) in (\"\")"=w206) -> ("States Out"=w205:string)  [unwired: 14 in]
      }
      frame "UI: Front Panel State" {
        # "Argument"
        # "Set Front Panel Open or Closed\n(Usage: \"UI: Front Panel State >> Open|Close\")"
        n75 = Unbundle By Name(w213) -> ("Core.Current VI Reference"=w212:refnum<vi>)
        n76 = case shown="\"Open\", Default" w211 {
          tunnel: w215 -> [w221 w234]
          tunnel: [w223 w235] -> w214
          tunnel: w212 -> [w222 w232]
          frame "Open", Default {
            n77 = property class="VI"(reference=w222, error in=w221) -> (reference out=w219:refnum<vi>, error out=w220:errorcluster, "Front Panel.Open"=w218:bool)
            n78 = case shown="False" w218 {
              tunnel: [w226 w229] -> w223
              tunnel: w220 -> [w225 w229]
              tunnel: w219 -> [w224 _]
              frame False {
                n79 = invoke class="VI" method="FP.Open"(reference=w224, error in=w225, "Activate"=TRUE, "State"=T10."Standard") -> (error out=w226:errorcluster)  [unwired: 1 in, 4 out]
              }
              frame True {
              }
            }
          }
          frame "Close" {
            n80 = property class="VI"(reference=w232, error in=w234) -> (reference out=w231:refnum<vi>, error out=w233:errorcluster, "Front Panel.Open"=w230:bool)
            n81 = case shown="True" w230 {
              tunnel: [w236 w239] -> w235
              tunnel: w233 -> [w236 w238]
              tunnel: w231 -> [_ w237]
              frame False {
              }
              frame True {
                n82 = invoke class="VI" method="FP.Close"(reference=w237, error in=w238) -> (error out=w239:errorcluster)  [unwired: 1 in, 2 out]
              }
            }
          }
        }
        n83 = call <vilib>:"Add State(s) to Queue__jki_lib_state_machine.vi"("State(s) in (\"\")"=w217) -> ("States Out"=w216:string)  [unwired: 14 in]
      }
      frame "---------- Macro ----------" {
        # "Do not put any code in this frame.\n(It is a separator no-op. You can make a copy of this frame to create a new Macro frame)"
        n84 = call <vilib>:"Add State(s) to Queue__jki_lib_state_machine.vi"("State(s) in (\"\")"=w243) -> ("States Out"=w242:string)  [unwired: 14 in]
      }
      frame "Macro: Initialize" {
        w244 = "Data: Initialize\nInitialize Core Data\nUI: Initialize\nUI: Front Panel State >> Open\nInit Draw"  # Data: Initialize Initialize Core Data UI: Initialize UI: Front Panel State >> Open Init Draw
        # "Initialization Macro\n(This is called once, when the VI starts)"
        n85 = call <vilib>:"Add State(s) to Queue__jki_lib_state_machine.vi"("State(s) in Front (\"\")"=w244, "State(s) in (\"\")"=w248) -> ("States Out"=w247:string)  [unwired: 13 in]
      }
      frame "Macro: Exit" {
        # "Exit Macro\n(This is called once, when the VI exits)"
        n86 = Unbundle By Name(w255) -> ("Core.Close Panel on Exit?"=w254:bool)
        n87 = Select(t="UI: Front Panel State >> Close", s=w254, f="") -> (s? t:f=w251:string)
        n88 = call <vilib>:"Add State(s) to Queue__jki_lib_state_machine.vi"("State(s) in (\"\")"=w251, "State(s) at Back (\"\")"="Data: Cleanup\nExit") -> ("States Out"=w249:string)  [unwired: 13 in]
        n89 = call <vilib>:"Add State(s) to Queue__jki_lib_state_machine.vi"("State(s) in Front (\"\")"=w249, "State(s) in (\"\")"=w258) -> ("States Out"=w257:string)  [unwired: 13 in]
      }
      frame "---------- New Category ----------" {
        # "Template Separator\n(You can make a copy of, or modify, this frame)"
        n90 = call <vilib>:"Add State(s) to Queue__jki_lib_state_machine.vi"("State(s) in (\"\")"=w262) -> ("States Out"=w261:string)  [unwired: 14 in]
      }
      frame "Init Draw" {
        w283 = T23 36 items=["4-20_OUT", "Pres_HI1", "Pres_HI2", "Pres_LOW", "Pres_PIN", "HEATER_TOP", "HEATER_BOT", "T_Shell", "FLOWMETER", "WATT_SENSE", "WH_TICK", "Tc_1", "Tc_2", "Tc_3", "Tc_4", "Tc_5", "Tc_6", "Tc_down", "T_Shell_2", "T_Shell_3", "T_Shell_4", "RTD_IN", "RTD_OUT", "RTD_AMB", "INTF_TEMPFLO", "INTF_READY", "INTF_START", "INTF_STOP", "DRM_LOW", "DRM_HIGH", "PWR_MAIN", "VLV_DUMP", "VLV_OUT", "VLV_IN", "WATT_HOURS", "FLOW(SAMPLE)", "GALLONS", "FLOW(GPM)"] ("Channel_Enum")
        # "AntiWaterHamer"
        n91 = Unbundle By Name(w265) -> ("Equipment.MW100"=w268:refnum<visa-resource-name>)
        n92 = call "Intellifaucet_Driver.vi"("VISA session"=w268, "Mode"=Intellfaucet_Mode."Stop Flow", "Error In"=w267) -> ("VISA session out"=w275:refnum<visa-resource-name>, "Error Out"=w272:errorcluster)  [unwired: 11 in]
        n93 = call "Solenoid - DRAIN.vi"("Error In"=w272, "VALVE OPEN CLOSE"=enum8{"OPEN", "CLOSE"}."CLOSE", "VISA session"=w275) -> ("Error Out"=w280:errorcluster, "dup VISA session"=w277:refnum<visa-resource-name>)  [unwired: 7 in]
        n94 = call "Solenoid - Fill.vi"("Error In"=w280, "VALVE OPEN CLOSE"=enum8{"OPEN", "CLOSE"}."OPEN", "VISA session"=w277) -> ("Error Out"=w279:errorcluster, "dup VISA session"=w278:refnum<visa-resource-name>)  [unwired: 7 in]
        n95 = call "Solenoid - Output_Set COM1 Val.vi"("Error In"=w279, "OPEN CLOSE"=enum8{"CLOSE", "OPEN"}."OPEN", "VISA session"=w278) -> ("Error Out"=w271:errorcluster, "dup VISA session"=w284:refnum<visa-resource-name>)  [unwired: 7 in]
        n96 = call "Delay mS.vi"("Error In"=w271, "milliseconds to wait"=u32 3000) -> ("Error Out"=w270:errorcluster)  [unwired: 13 in]
        n97 = call "Intellifaucet_Driver.vi"("VISA session"=w284, "Mode"=Intellfaucet_Mode."Start Flow", "Error In"=w270) -> ("VISA session out"=w282:refnum<visa-resource-name>, "Error Out"=w285:errorcluster)  [unwired: 11 in]
        n98 = call "E-Time.vi"("error in (no error)"=w285) -> ("error out"=w281:errorcluster, "Elapsed Time (sec)"=→"Current Draw Start Time":dbl)  [unwired: 8 in, 1 out]
        n99 = call "Generic - AI1.vi"("MW100"=w282, "Channel_Enum"=w283, "Error In"=w281) -> ("Value"=w263:dbl, "Error Out"=w266:errorcluster)  [unwired: 10 in, 1 out]
        n100 = Bundle By Name(cluster=w265, "Start Gallons"=w263) -> (w264:T21)
        n101 = call <vilib>:"Add State(s) to Queue__jki_lib_state_machine.vi"("State(s) in (\"\")"=w290) -> ("States Out"=w289:string)  [unwired: 14 in]
      }
      frame "Gather Data" {
        n102 = Unbundle By Name(w299) -> ("Equipment"=w303:T3, "User Controls.GEA2?"=w302:bool, "FileInit Cluster.Calibration Coefficients"=w300:dbl[][])
        n103 = local read "Elapsed Time"() -> (w293:T2)
        n104 = call "E-Time.vi"("error in (no error)"=w296) -> ("error out"=w295:errorcluster, "Elapsed Time (sec)"=w294:dbl)  [unwired: 8 in, 1 out]
        "Gather Data Timer" <- w294
        n105 = Subtract(x=w294, y=w293) -> (x-y=→"Loop Time":T2)
        n106 = control-ref of="Tank Display"() -> (w304:refnum<vi>)
        n107 = call "Gather Test Data - Heatup Test new.vi"("GEA2?"=w302, "Equipment"=w303, "Tank Display Ref"=w304, "Calibration Coefficients"=w300, "error in (no error)"=w295) -> ("PowerData"=w297:T1, "error out"=w301:errorcluster)  [unwired: 6 in, 3 out]
        "PowerData" <- w297
        n108 = Unbundle By Name(w297) -> ("Flow Rate (GPM)"=→"Flow Chart":dbl)
        n109 = Bundle By Name(cluster=w299, "PowerData"=w297) -> (w298:T21)
        n110 = call <vilib>:"Add State(s) to Queue__jki_lib_state_machine.vi"("State(s) in (\"\")"=w306) -> ("States Out"=w305:string)  [unwired: 14 in]
      }
      frame "Init Set Flow" {
        # "You have to run a calibration procedure\non the intellifaucet before this is fast as \npossible. It then takes and interpolates\nthose values for the quickest initial setpoint"
        # "Allows the flow to stabilize before the \nPID loop kicks in. This routine allows \nfor quicker startup times"
        n111 = Unbundle By Name(w315) -> ("Equipment.MW100"=w309:refnum<visa-resource-name>, "PowerData.Flow Rate (GPM)"=w308:dbl, "GPM Target Value"=w307:dbl)
        n112 = local read "Configuration"() -> (w311:T5)
        n113 = call "Linear Interpolation GPM to Percent Open.vi"("Interp Direction"=enum16{"GPM to Percent", "Percent to GPM"}."GPM to Percent", "Input (GPM,Percent)"=w307, "Configuration"=w311) -> ("Output (Percent,GPM)"=w312:dbl)  [unwired: 8 in]
        n114 = call "Intellifaucet_Driver.vi"("VISA session"=w309, "Mode"=Intellfaucet_Mode."Adjust Flow", "Percent Flow"=w312, "Error In"=w313) -> ("Error Out"=w317:errorcluster)  [unwired: 10 in, 1 out]
        n115 = Bundle By Name(cluster=w315, "Last GPM Reading"=w308) -> (w316:T21)
        n116 = call <vilib>:"Add State(s) to Queue__jki_lib_state_machine.vi"("State(s) in (\"\")"=w319) -> ("States Out"=w318:string)  [unwired: 14 in]
      }
      frame "Adjust Flow" {
        n117 = local read "Current Draw Start Time"() -> (w332:dbl)
        n118 = Unbundle By Name(w323) -> ("Equipment.MW100"=w339:refnum<visa-resource-name>, "GPM Target Value"=w335:dbl, "PowerData.Flow Rate (GPM)"=w338:dbl, "Last GPM Reading"=w337:dbl, "PowerData.Gallons (Gal)"=w331:dbl, "Start Gallons"=w330:dbl, "Gallon Target Value"=w328:dbl)
        n119 = call "E-Time.vi"("error in (no error)"=w334) -> ("error out"=w333:errorcluster, "Elapsed Time (sec)"=w324:dbl)  [unwired: 8 in, 1 out]
        n120 = Subtract(x=w331, y=w330) -> (x-y=w329:dbl)
        "Dispensed Gallons" <- w329
        n121 = Subtract(x=w324, y=w332) -> (x-y=→"Elapsed Time":dbl)
        n122 = call "HEWH Flow Adjustment.vi"("VISA session"=w339, "Configuration"="Configuration", "GPM Target(3)"=w335, "GPM reading"=w338, "New GPM Reading \nfrom last adjustment"=w337, "Error In"=w333) -> ("Flow rate setting Out"=w321:dbl, "Error Out"=w320:errorcluster)  [unwired: 7 in, 1 out]
        n123 = Greater Or Equal?(x=w329, y=w328) -> (x >= y?=w326:bool)
        n124 = Bundle By Name(cluster=w323, "Last GPM Reading"=w321) -> (w322:T21)
        n125 = case shown="False" w326 {
          tunnel: ["" "Term Draw\nMacro: Exit"] -> w325
          frame False {
          }
          frame True {
          }
        }
        n126 = call <vilib>:"Add State(s) to Queue__jki_lib_state_machine.vi"("State(s) in Front (\"\")"=w325, "State(s) in (\"\")"=w341) -> ("States Out"=w340:string)  [unwired: 13 in]
      }
      frame "Term Draw" {
        # "Must allow time for I.F. to close all the way."
        # "Keep line pressure on tank."
        n127 = Unbundle By Name(w345) -> ("Equipment.MW100"=w344:refnum<visa-resource-name>)
        n128 = call "Intellifaucet_Driver.vi"("VISA session"=w344, "Mode"=Intellfaucet_Mode."Stop Flow", "Error In"=w347) -> ("Error Out"=w350:errorcluster)  [unwired: 11 in, 1 out]
        n129 = call "Delay mS.vi"("Error In"=w350, "milliseconds to wait"=u32 500) -> ("Error Out"=w351:errorcluster)  [unwired: 13 in]
        n130 = call "Solenoid - Output_Set COM1 Val.vi"("Error In"=w351, "OPEN CLOSE"=enum8{"CLOSE", "OPEN"}."CLOSE") -> ("Error Out"=w355:errorcluster)  [unwired: 8 in, 1 out]
        n131 = call "Delay mS.vi"("Error In"=w355, "milliseconds to wait"=u32 2500) -> ("Error Out"=w356:errorcluster)  [unwired: 13 in]
        n132 = call "Intellifaucet_Driver.vi"("VISA session"=w344, "Mode"=Intellfaucet_Mode."Start Flow", "Error In"=w356) -> ("Error Out"=w346:errorcluster)  [unwired: 11 in, 1 out]
        n133 = call <vilib>:"Add State(s) to Queue__jki_lib_state_machine.vi"("State(s) in (\"\")"=w358) -> ("States Out"=w357:string)  [unwired: 14 in]
      }
    }
  }
